vi "endTime.get.vi"(8 "error in (no error)":errorcluster, 11 "Run in":refnum<class "Run.lvclass">) -> (0 "error out":errorcluster, 2 "endTime":timestamp format="%<%x %.3X>T", 3 "Run out":refnum<class "Run.lvclass">)   [LabVIEW 2020, in "Run.lvclass"]
uses:
  Run.lvclass
  Run.lvclass/Run.ctl
  3ccb7712-5e93-42a8-8ce3-daf6d605bb4c.vi
  <vilib>/LabVIEW Open Source Project/Epoch Date & Time/epoch.UNIX/Epoch.UNIX.lvclass
  999315d3-869a-4829-82f3-8c20d3f4bab2.vi
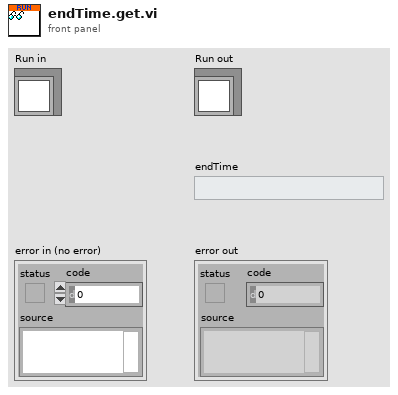
[diagram p1: front panel]
types:
  T1 = cluster{"secondsSinceEpoch":i32, "offsetNanoseconds":i32}
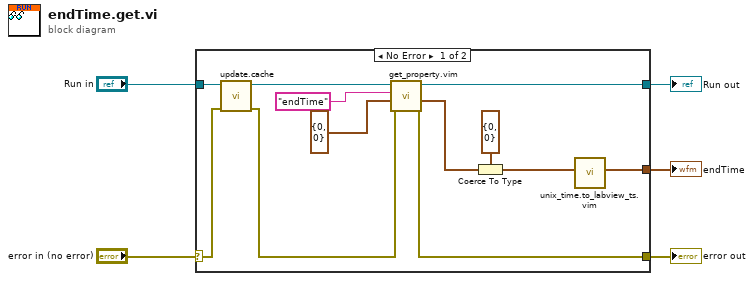
[diagram p0: block diagram]
diagram:
  n1 = case shown="No Error" "error in (no error)" {
    selector: "error in (no error)" -> [w17 w18]
    tunnel: [w6 w18] -> w4
    tunnel: [w11 w19] -> w2
    tunnel: "Run in" -> [w15 w19]
    tunnel: [w16 _] -> w1
    frame No Error {
      n2 = call "update.cache.vi"("error in"=w17, "Run in"=w15) -> ("error out"=w7:errorcluster, "Run out"=w12:refnum<class "Run.lvclass">)  [unwired: 8 in]
      n3 = call "get_property.vim"("error in"=w7, "default value and type"=T1 {"secondsSinceEpoch"=0, "offsetNanoseconds"=0} ("endTime"), "Property Name"="endTime", "Run in"=w12) -> ("error out"=w6:errorcluster, "Value"=w10:T1, "Run out"=w11:refnum<class "Run.lvclass">)  [unwired: 5 in]
      n4 = Coerce To Type(0:w10, 1:cluster{"Seconds":i32, "Nanoseconds":i32} {"Seconds"=0, "Nanoseconds"=0} ("UNIX Timestamp")) -> (2:w8:cluster{"Seconds":i32, "Nanoseconds":i32})
      n5 = call "unix_time.to_labview_ts.vim"("UNIX Timestamp"=w8) -> ("Time Stamp"=w16:timestamp)  [unwired: 10 in]
    }
    frame Error {
    }
  }
  "error out" <- w4
  "Run out" <- w2
  "endTime" <- w1
